vi "Get Username.vi"(8 "error in (no error)":errorcluster, 10 "User Level":enum16{"Administrator", "Engineer", "Operator"}(ring), 11 "MySQL in":refnum<class "MySQL.lvclass">) -> (0 "error out":errorcluster, 2 "Username":string[](array[string]), 3 "MySQL out":refnum<class "MySQL.lvclass">)   [LabVIEW 2021, in "Database.lvlib" / "MySQL.lvclass"]
uses:
  MySQL.lvclass
  MySQL.lvclass/MySQL.ctl
  <vilib>/addons/database/NI_Database_API.lvlib
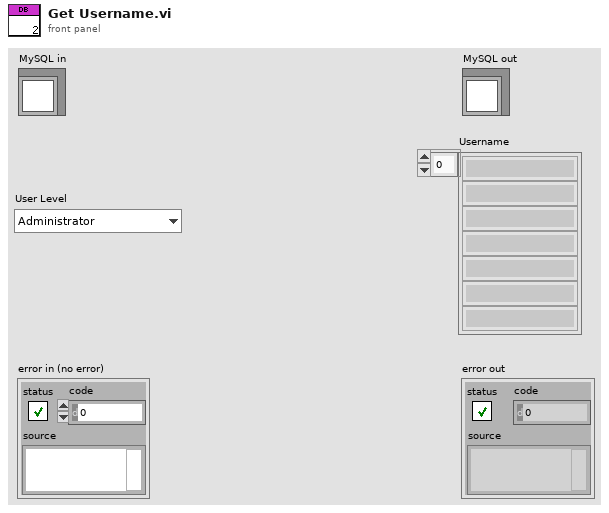
[diagram p1: front panel]
types:
  T1 = typedef "Database.lvlib/DB.lvclass/Table_info.ctl" = cluster{"Authentication":string, "Instr_Configuration":string, "Recipe":string, "Test_data":string}
  T2 = typedef "NI_Database_API.lvlib/Conn ObjectReference.ctl" = refnum<k1>
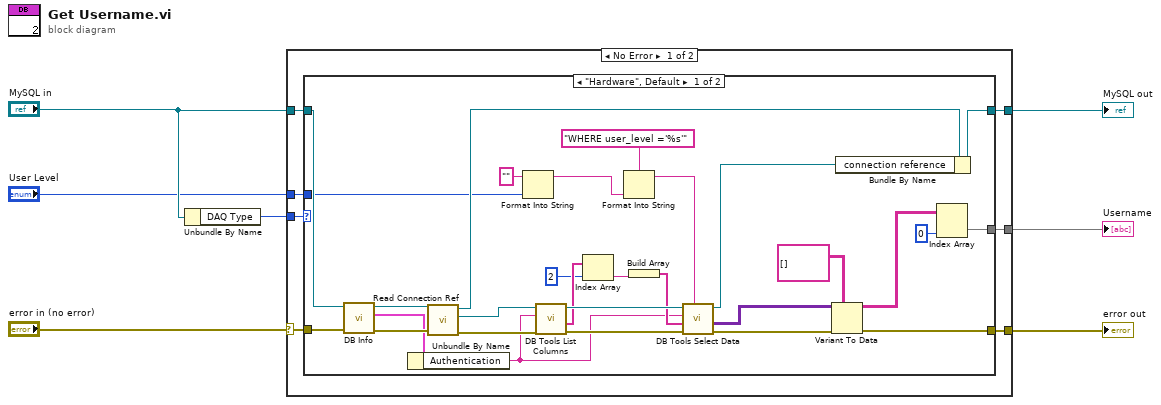
[diagram p0: block diagram]
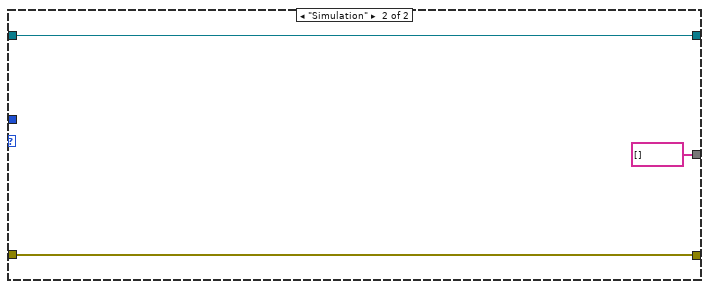
[diagram p2: hidden frame]
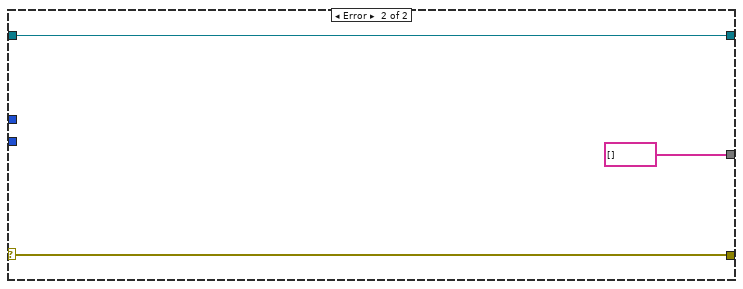
[diagram p3: hidden frame]
diagram:
  n1 = Unbundle By Name("MySQL in") -> ("DAQ Type"=w7:enum16{"Hardware", "Simulation"})
  n2 = case shown="No Error" "error in (no error)" {
    selector: "error in (no error)" -> [w14 w48]
    tunnel: "MySQL in" -> [w13 w49]
    tunnel: [w12 w48] -> w1
    tunnel: [w11 w49] -> w3
    tunnel: [w10 string[] []] -> w2
    tunnel: "User Level" -> [w9 _]
    tunnel: w7 -> [w8 _]
    frame No Error {
      n3 = case shown="\"Hardware\", Default" w8 {
        tunnel: w14 -> [w43 w45]
        tunnel: w13 -> [w42 w46]
        tunnel: [w26 w45] -> w12
        tunnel: [w24 w46] -> w11
        tunnel: [w20 string[] []] -> w10
        tunnel: w9 -> [w18 _]
        frame "Hardware", Default {
          n4 = call-dynamic "DB Info.vi"("error in (no error)"=w43, "MySQL in"=w42) -> ("error out"=w40:errorcluster, "Table_info"=w29:T1, "MySQL out"=w41:refnum<class "MySQL.lvclass">)  [unwired: 6 in, 1 out]
          n5 = Unbundle By Name(w29) -> ("Authentication"=w28:string)
          n6 = call-dynamic "Read Connection Ref.vi"("error in (no error)"=w40, "MySQL in"=w41) -> ("error out"=w34:errorcluster, "connection reference"=w35:T2, "MySQL out"=w25:refnum<class "MySQL.lvclass">)  [unwired: 7 in]
          n7 = Format Into String(initial string="", w18) -> (resulting string=w16:string)  [unwired: 2 in, 1 out]
          n8 = call <vilib>:"DB Tools List Columns.vi"("error in (no error)"=w34, "table"=w28, "connection reference"=w35) -> ("error out"=w39:errorcluster, "columns"=w33:string[], "connection reference out"=w38:T2)  [unwired: 1 in, 1 out]
          n9 = Index Array(array=w33, index=2) -> (element=w31:string)
          n10 = Format Into String(format string="WHERE user_level ='%s'" ("condition"), w16) -> (resulting string=w15:string)  [unwired: 2 in, 1 out]
          n11 = Build Array(w31) -> (w30:string[])
          n12 = call <vilib>:"DB Tools Select Data.vi"("condition"=w15, "error in (no error)"=w39, "columns"=w30, "table"=w28, "connection reference"=w38) -> ("error out"=w37:errorcluster, "data"=w27:variant[][], "connection reference out"=w23:T2)  [unwired: 1 in]
          n13 = Variant To Data(error in=w37, type=string[][] [], Variant=w27) -> (data=w22:string[][], error out=w26:errorcluster)
          n14 = Bundle By Name(cluster=w25, "connection reference"=w23) -> (w24:refnum<class "MySQL.lvclass">)
          n15 = Index Array(array=w22, index (col)=0 ("disabled index (col)")) -> (element=w20:string[])  [unwired: 1 in]
        }
        frame "Simulation" {
        }
      }
    }
    frame Error {
    }
  }
  "error out" <- w1
  "MySQL out" <- w3
  "Username" <- w2
